vi "tmp.vi"(8 "error in (no error)":errorcluster, 10 "fun2call":T1, 11 "Arguments":cluster{"arg1":i32, "arg2":dbl}) -> (0 "error out":errorcluster, 3 "JSON string":string)   [LabVIEW 2018, in "LV-Julia_ZMQ-Roundtrip_lib.lvlib"]
uses:
  LV-Julia_ZMQ-Roundtrip_lib.lvlib
  Julia functions enum.ctl
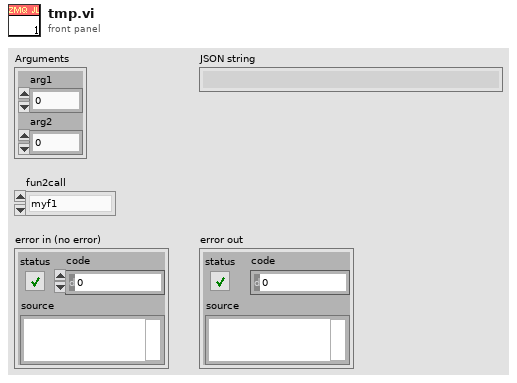
[diagram p1: front panel]
types:
  T1 = typedef "LV-Julia_ZMQ-Roundtrip_lib.lvlib/Julia functions enum.ctl" = enum16{"myf1", "myf2", "myf3", "bin2num"}
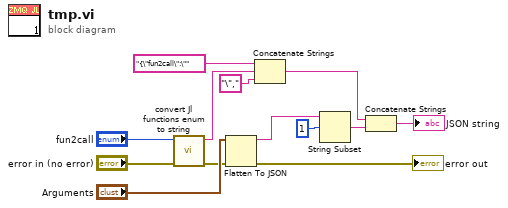
[diagram p0: block diagram]
diagram:
  n1 = call "convert Jl functions enum to string.vi"("error in (no error)"="error in (no error)", "fun2call"="fun2call") -> ("error out"=w6:errorcluster, "String out"=w5:string)  [unwired: 8 in]
  n2 = Flatten To JSON(anything="Arguments", error in (no error)=w6) -> (JSON string=w12:string, 11:→"error out":errorcluster)  [unwired: 1 in]
  n3 = Concatenate Strings("{\"fun2call\":\"" ("string"), w5, "\"," ("string")) -> (w1:string)
  n4 = String Subset(string=w12, offset (0)=1) -> (substring=w13:string)  [unwired: 1 in]
  n5 = Concatenate Strings(w1, w13) -> (→"JSON string":string)
